vi "TEST.vi"() -> ()   [LabVIEW 2009, in "Servo.lvlib"]
uses:
  Servo.lvlib
  PWM/PWM_Name.ctl
  PWM.lvlib
panel:
  out "unsigned 32bit integer":u32
  out "FPGA_Ref_out":refnum<k20>
  in  "FPGA_Ref_in":refnum<k20>
  out "error out":errorcluster
  in  "error in":errorcluster
  in  "y":dbl
  in  "x":dbl min=-45.0 max=45.0
  in  "PWM":T1=1 items=["Invalid"=0, "PWM1"=1, "PWM2"=2, "PWM9"=9, "PWM10"=10]
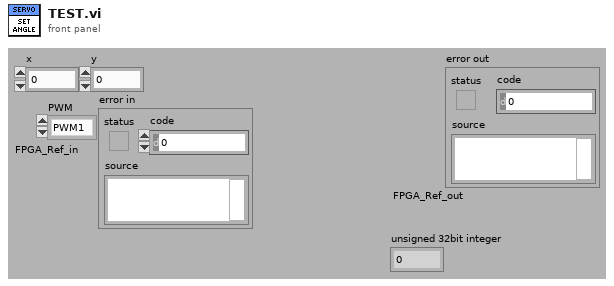
[diagram p1: front panel]
types:
  T1 = typedef "PWM.lvlib/PWM_Name.ctl" = u16
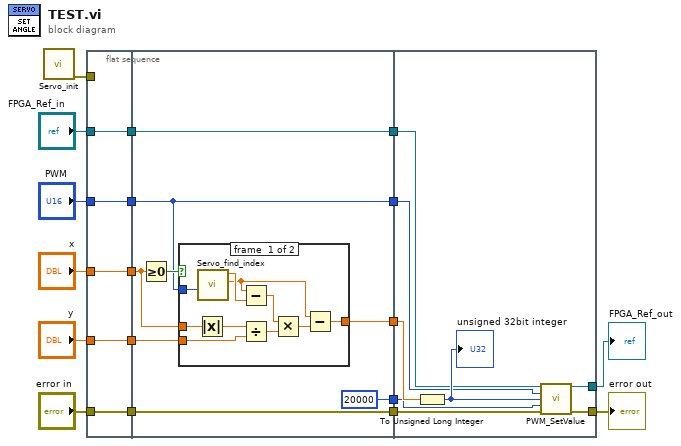
[diagram p0: block diagram]
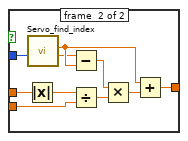
[diagram p2: hidden frame]
diagram:
  n1 = call "Servo_init.vi"() -> ("error out"=w17:errorcluster)  [unwired: 11 in]
  n2 = flat-sequence {
    tunnel: "PWM" -> [w22]
    tunnel: w17 -> [_]
    tunnel: "x" -> [w23]
    tunnel: [w23] -> w15
    tunnel: [w22] -> w14
    tunnel: "y" -> [w21]
    tunnel: [w21] -> w12
    tunnel: "error in" -> [w20]
    tunnel: [w20] -> w8
    tunnel: "FPGA_Ref_in" -> [w19]
    tunnel: [w19] -> w2
    tunnel: w15 -> [w30]
    tunnel: w14 -> [w25]
    tunnel: [w29] -> w13
    tunnel: w12 -> [w28]
    tunnel: [u32 20000 ("Period (uSec)")] -> w10
    tunnel: [w26] -> w9
    tunnel: w8 -> [w26]
    tunnel: [w25] -> w5
    tunnel: [w24] -> w3
    tunnel: w2 -> [w24]
    tunnel: w13 -> [w59]
    tunnel: w10 -> [w57]
    tunnel: w9 -> [w56]
    tunnel: [w55] -> w6
    tunnel: w5 -> [w54]
    tunnel: w3 -> [w53]
    tunnel: [w52] -> w1
    frame #0 {
    }
    frame #1 {
      n3 = Greater Or Equal To 0?(x=w30) -> (x >= 0?=w31:bool)
      n4 = case shown="True" w31 {
        tunnel: w30 -> [w40 w50]
        tunnel: w25 -> [w41 w51]
        tunnel: [w37 w45] -> w29
        tunnel: w28 -> [w33 w47]
        frame #0 {
          n5 = Absolute Value(x=w40) -> (abs(x)=w34:dbl)
          n6 = call "Servo_find_index.vi"("PWM"=w41) -> ("value 2"=w35:dbl, "value"=w38:dbl)  [unwired: 7 in, 2 out]
          n7 = Subtract(x=w35, y=w38) -> (x-y=w39:dbl)
          n8 = Divide(x=w34, y=w33) -> (x/y=w32:dbl)
          n9 = Multiply(x=w39, y=w32) -> (x*y=w36:dbl)
          n10 = Subtract(x=w35, y=w36) -> (x-y=w37:dbl)
        }
        frame #1 {
          n11 = Absolute Value(x=w50) -> (abs(x)=w48:dbl)
          n12 = call "Servo_find_index.vi"("PWM"=w51) -> ("value 3"=w42:dbl, "value 2"=w43:dbl)  [unwired: 7 in, 2 out]
          n13 = Subtract(x=w42, y=w43) -> (x-y=w49:dbl)
          n14 = Divide(x=w48, y=w47) -> (x/y=w46:dbl)
          n15 = Multiply(x=w49, y=w46) -> (x*y=w44:dbl)
          n16 = Add(x=w43, y=w44) -> (x+y=w45:dbl)
        }
      }
    }
    frame #2 {
      n17 = To Unsigned Long Integer(number=w59) -> (unsigned 32bit integer=w58:u32)
      "unsigned 32bit integer" <- w58
      n18 = call "PWM_SetValue.vi"("FPGA_Ref_in"=w53, "PWM"=w54, "High (uSec)"=w58, "Period (uSec)"=w57, "error in"=w56) -> ("FPGA_Ref_out"=w52:refnum<k20>, "error out"=w55:errorcluster)  [unwired: 9 in]
    }
  }
  "error out" <- w6
  "FPGA_Ref_out" <- w1
